vi "New if invalid.vi"(8 "error in (no error)":errorcluster, 11 "Signaller in":refnum<class "Signaller.lvclass">) -> (0 "error out":errorcluster, 3 "Signaller out":refnum<class "Signaller.lvclass">)   [LabVIEW 2019, in "Signaller.lvclass"]
uses:
  Signaller.lvclass
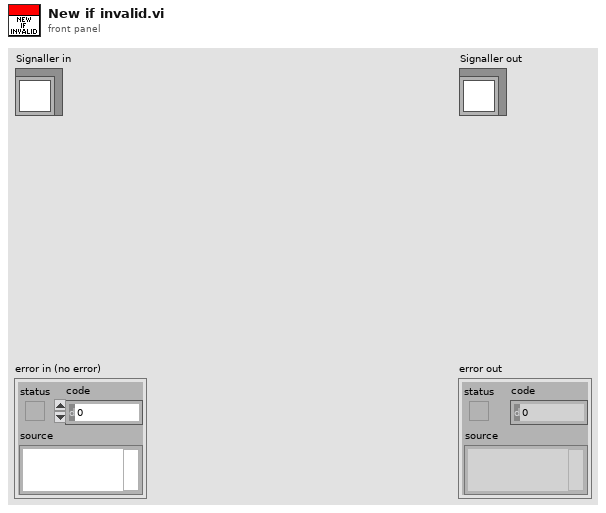
[diagram p1: front panel]
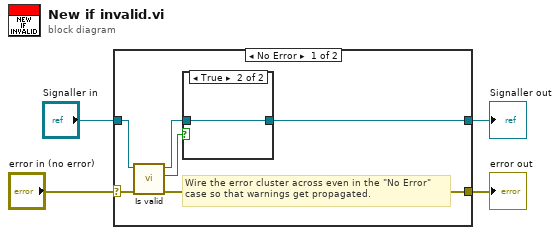
[diagram p0: block diagram]
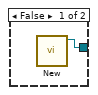
[diagram p2: hidden frame]
diagram:
  n1 = case shown="No Error" "error in (no error)" {
    selector: "error in (no error)" -> [w8 w14]
    tunnel: [w7 w14] -> w3
    tunnel: [w10 w13] -> w1
    tunnel: "Signaller in" -> [w9 w13]
    frame No Error {
      # "Wire the error cluster across even in the \"No Error\"\ncase so that warnings get propagated."
      n2 = call "Is valid.vi"("error in (no error)"=w8, "Signaller in"=w9) -> ("error out"=w7:errorcluster, "Is valid?"=w6:bool, "Signaller out"=w5:refnum<class "Signaller.lvclass">)  [unwired: 7 in]
      n3 = case shown="True" w6 {
        tunnel: [w11 w12] -> w10
        tunnel: w5 -> [_ w12]
        frame False {
          n4 = call "New.vi"() -> ("Signaller out"=w11:refnum<class "Signaller.lvclass">)  [unwired: 11 in]
        }
        frame True {
        }
      }
    }
    frame Error {
    }
  }
  "error out" <- w3
  "Signaller out" <- w1
